vi "Assert 64 bit wired to 64 bit Type.vi"   [LabVIEW 2017]
uses:
  db8402c5-9e09-4326-9251-2cdded9c337c.vi
  a3e51480-a4f9-474e-88e9-58ae78dca282.vi
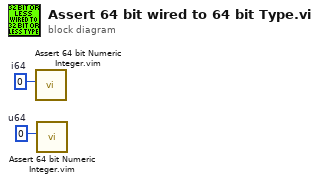
[diagram p0: block diagram]
diagram:
  w1 = i64 0  # i64
  w2 = u64 0  # u64
  n1 = call "Assert 64 bit Numeric Integer.vim"("Item in"=w1) -> ()  [unwired: 10 in, 1 out]
  n2 = call "Assert 64 bit Numeric Integer.vim"("Item in"=w2) -> ()  [unwired: 10 in, 1 out]
